vi "_read_LO_params.vi"(10 "Control":T5={"GPIB_ATT"="28", "6501Dev#"=1, "GPIB_SP"="18", "GPIB_PM"="13", "GPIB_DSA"="11", "GPIB_DMM (TPD)"="23", "GPIB_MPI"="2", "mortorÝè"=[{"Axis"=0, "ID"=0, "HIspeed"=200.0, "LOspeed"=100.0, "ACCEL(ms)"=100.0, "Sratio"=50.0, "フリーラン\n"=FALSE, "•¶Žš—ñ"="DSB HOT/COLD"}, {"Axis"=1, "ID"=0, "HIspeed"=4.0, "LOspeed"=4.0, "ACCEL(ms)"=100.0, "Sratio"=50.0, "フリーラン\n"=TRUE, "•¶Žš—ñ"="SubMM Att"}, {"Axis"=0, "ID"=0, "HIspeed"=200.0, "LOspeed"=100.0, "ACCEL(ms)"=100.0, "Sratio"=50.0, "フリーラン\n"=TRUE, "•¶Žš—ñ"="MPI Port1"}, {"Axis"=1, "ID"=0, "HIspeed"=200.0, "LOspeed"=100.0, "ACCEL(ms)"=100.0, "Sratio"=50.0, "フリーラン\n"=TRUE, "•¶Žš—ñ"="MPI Port2"}, {"Axis"=1, "ID"=0, "HIspeed"=200.0, "LOspeed"=100.0, "ACCEL(ms)"=100.0, "Sratio"=50.0, "フリーラン\n"=TRUE, "•¶Žš—ñ"="gainComp"}], "DATAパス"=path "C:/Documents and Settings/?澤佳?/デスクトップ/data/プロトカ?トリッジ/110113_protoC4-9/110127_mixtest", "DBパス "=path "Z:/band10/Labview_ALMA/MIX95/test", "comment"="mix10test", "ColdCarts"="003601", "Th"=300.0, "Tc"=77.0, "Set_SIS_volt"=2.0999999046325684, "Offset"=0.0, "control"=0, "FreqLO"=874.0, "Set_Mag_Cur"=800.0, "MPI offset(mm)"=22.962, "HOT/COLD"=0} {"HOT/COLD" items=["DSB", "SBR (Cart.)", "GainComp", "SBR (MIX)"]; "control" items=["CLOSE LOOP", "OPEN LOOP", "Not Control"]}, 11 "Bias_LO_equip":T7={"Node address"=19, "CAN Interface"="CAN1", "Cartridge band"=10, "Slave Node in"={"Address"=19, "Serial Number"=[16, 71, 55, 76, 1, 8, 0, -15]}, "ObjHandle out"=214106176, "POL"=1, "sb"=1, "GPIB_SM (SIS S,V)"="24", "GPIB_DMM (SIS I)"="22", "GPIB_SM (MAG I) "="25", "GPIB_SG(LO)"="19", "GPIB_PW (PAMP) "="6", "GPIB_TMP1(8ch)"="12", "GPIB_TMP2(2ch)  "="13", "WCA_avg"=10, "Rsen"=10.0, "BiasModule"=1, "LOModule "=5, "WCA_LO_FREQ_SET"={"YTO Low freq. [GHz]"=14.42, "YTO High freq. [GHz]"=17.7, "Kvco"=1, "Lock Pol."=0, "SET LO FREQ"=96.22222, "Multiplier"=6.0, "YTO (HEX)"=2014, "YTO ( FREQ)"=16.033167, "NULL PLL INTEGRATOR"=FALSE}, "Res for"=0} {"Res for" items=["none", "series res", "parallel res"]; "WCA_LO_FREQ_SET"."YTO ( FREQ)" min=25 max=150 step=0.0001 format="%.3f"; "WCA_LO_FREQ_SET"."Multiplier" min=3 max=6 step=3; "WCA_LO_FREQ_SET"."SET LO FREQ" min=25 max=150 step=0.0001 format="%.3f"; "WCA_LO_FREQ_SET"."Lock Pol." items=["Lower", "Upper"]; "WCA_LO_FREQ_SET"."Kvco" items=["7.5MHz/V", "15MHz/V"]; "WCA_LO_FREQ_SET"."YTO High freq. [GHz]" format="%.3f"; "WCA_LO_FREQ_SET"."YTO Low freq. [GHz]" format="%.3f"; "BiasModule" items=["B10Lab Bias"=0, "WCA BiasModule"=1, "none"=99]; "Slave Node in"."Serial Number" format="%.0x"; "Slave Node in"."Address" format="%.0x"; "Cartridge band" max=10 step=1; "Node address" format="%.0x"}) -> (3 "•¶Žš—ñ":string="PreampParam, 3.65, 874.00, 2011-02-04  19:50:11, 1.40, 0.00, 0.00,  12.05, 0.00, 0.02,  -1.53, 4.91, 4.91,")   [LabVIEW 2017]
uses:
  WCA_NAOJ_sub_vi/WCA_Global.vi
panel:
  out "GET_PLL":T1={"PLL_ASSY_T"=37.887573, "PLL_REF_TOT_P"=-0.004119873, "PLL_IF_TOT_P"=0.010223389, "PLL_CORR_V"=0.08273038, "PLL_LOCK_V"=0.06496083, "PLL_5V_SUPPLY_V"=19.049072, "Temp_TF"=TRUE, "PLL Ref Pwr_TF"=FALSE, "IF Pwr_TF"=FALSE, "PLL Corr_TF"=TRUE, "PLL Lock V_TF"=FALSE, "PLL Nominal_TF"=FALSE}
  out "GET_PA":T2={"PA_A_DRAIN_V"=4.0403748, "PA_A_DRAIN_C"=429.99268, "PA_A_GATE_V"=-0.00061035156, "PA_B_DRAIN_V"=0.0048828125, "PA_B_DRAIN_C"=2.5482178, "PA_B_GATE_V"=0.0015258789, "PA_3V_SUPPLY_V"=3.7130737, "PA_5V_MON"=5.3082275}
  out "GET_AMC":T3={"AMC_A_DRAIN_V"=3.48938, "AMC_A_DRAIN_C"=64.42261, "AMC_A_GATE_V"=-0.4689026, "AMC_B_DRAIN_V"=4.34021, "AMC_B_DRAIN_C"=301.4679, "AMC_B_GATE_V"=-0.48934937, "AMC_E_DRAIN_V"=3.977356, "AMC_E_DRAIN_C"=342.6819, "AMC_E_GATE_V"=-0.24169922, "AMC_3V_SUPPLY_V"=-13.227844, "AMC_5V_MON"=5.204468, "AMC_MULT_D_V"=0.0}
  out "GET_PHOTOMIXER":T4={"PHOTMIX_ State"=enum."Disabled", "PHOTOMIX_BIAS_V"=-0.0012207031, "PHOTOMIX_BIAS_C"=-0.0032043457}
  in  "CLNA_SET":T6={"CLNA State"=1, "SET POL0 LNA1 STAGE1 DRAIN V"=0.0, "SET POL0 LNA1 STAGE1 DRAIN C"=0.0, "SET POL0 LNA1 STAGE2 DRAIN V"=0.0, "SET POL0 LNA1 STAGE2 DRAIN C"=0.0, "SET POL0 LNA1 STAGE3 DRAIN V"=0.0, "SET POL0 LNA1 STAGE3 DRAIN C"=0.0} {"SET POL0 LNA1 STAGE3 DRAIN C" min=0 max=20 step=0.01 format="%.2f"; "SET POL0 LNA1 STAGE3 DRAIN V" min=0 max=3 step=0.01 format="%.2f"; "SET POL0 LNA1 STAGE2 DRAIN C" min=0 max=20 step=0.01 format="%.2f"; "SET POL0 LNA1 STAGE2 DRAIN V" min=0 max=3 step=0.01 format="%.2f"; "SET POL0 LNA1 STAGE1 DRAIN C" min=0 max=20 step=0.01 format="%.2f"; "SET POL0 LNA1 STAGE1 DRAIN V" min=0 max=3 step=0.01 format="%.2f"; "CLNA State" items=["Disabled", "Enabled"]}
  out "Link済み":bool
  # "Vd [V]"
  # "Id [mA]"
  # "Vg [V]"
  # "PA -3V Supply"
  # "PA A"
  # "-3V"
  # "PA B"
  # "+5V"
  # "Vd [V]"
  # "Id [mA]"
  # "Vg [V]"
  # "AMC A"
  # "AMC B"
  # "AMC E"
  # "Vd [V]"
  # "Id [mA]"
  # "Stage 1"
  # "Stage 2"
  # "Stage 3"
  # "LO freq. [GHz]"
  # "YTO LOW\n/High Freq."
  # "ZERO Intgrtr"
  # "Node Address"
  # "Serial Number"
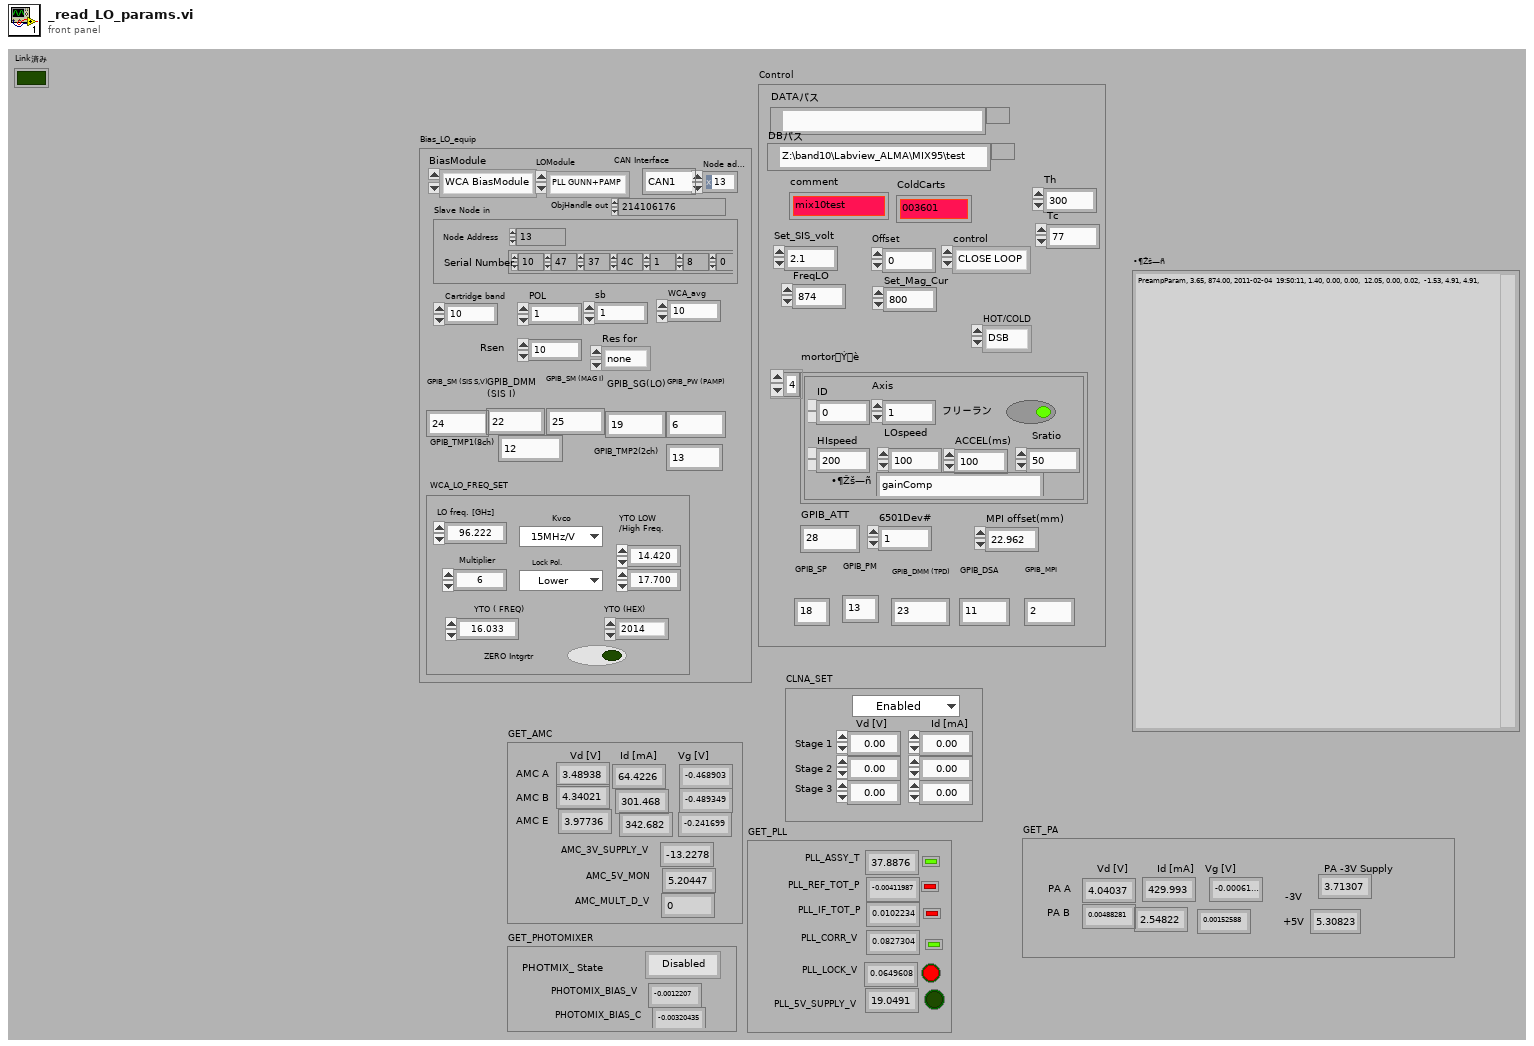
[diagram p1: front panel]
types:
  T1 = cluster{"PLL_ASSY_T":sgl, "PLL_REF_TOT_P":sgl, "PLL_IF_TOT_P":sgl, "PLL_CORR_V":sgl, "PLL_LOCK_V":sgl, "PLL_5V_SUPPLY_V":sgl, "Temp_TF":bool, "PLL Ref Pwr_TF":bool, "IF Pwr_TF":bool, "PLL Corr_TF":bool, "PLL Lock V_TF":bool, "PLL Nominal_TF":bool}
  T2 = cluster{"PA_A_DRAIN_V":sgl, "PA_A_DRAIN_C":sgl, "PA_A_GATE_V":sgl, "PA_B_DRAIN_V":sgl, "PA_B_DRAIN_C":sgl, "PA_B_GATE_V":sgl, "PA_3V_SUPPLY_V":sgl, "PA_5V_MON":sgl}
  T3 = cluster{"AMC_A_DRAIN_V":sgl, "AMC_A_DRAIN_C":sgl, "AMC_A_GATE_V":sgl, "AMC_B_DRAIN_V":sgl, "AMC_B_DRAIN_C":sgl, "AMC_B_GATE_V":sgl, "AMC_E_DRAIN_V":sgl, "AMC_E_DRAIN_C":sgl, "AMC_E_GATE_V":sgl, "AMC_3V_SUPPLY_V":sgl, "AMC_5V_MON":sgl, "AMC_MULT_D_V":sgl}
  T4 = cluster{"PHOTMIX_ State":enum16{"Disabled", "Enabled"}, "PHOTOMIX_BIAS_V":sgl, "PHOTOMIX_BIAS_C":sgl}
  T5 = cluster{"GPIB_ATT":string, "6501Dev#":i16, "GPIB_SP":string, "GPIB_PM":string, "GPIB_DSA":string, "GPIB_DMM (TPD)":string, "GPIB_MPI":string, "mortorÝè":cluster{"Axis":i16, "ID":i16, "HIspeed":dbl, "LOspeed":dbl, "ACCEL(ms)":dbl, "Sratio":dbl, "フリーラン\n":bool, "•¶Žš—ñ":string}[], "DATAパス":path, "DBパス ":path, "comment":string, "ColdCarts":string, "Th":dbl, "Tc":dbl, "Set_SIS_volt":dbl, "Offset":dbl, "control":u16, "FreqLO":dbl, "Set_Mag_Cur":dbl, "MPI offset(mm)":dbl, "HOT/COLD":u16}
  T6 = cluster{"CLNA State":u8, "SET POL0 LNA1 STAGE1 DRAIN V":sgl, "SET POL0 LNA1 STAGE1 DRAIN C":sgl, "SET POL0 LNA1 STAGE2 DRAIN V":sgl, "SET POL0 LNA1 STAGE2 DRAIN C":sgl, "SET POL0 LNA1 STAGE3 DRAIN V":sgl, "SET POL0 LNA1 STAGE3 DRAIN C":sgl}
  T7 = cluster{"Node address":u16, "CAN Interface":string, "Cartridge band":u32, "Slave Node in":cluster{"Address":i16, "Serial Number":i8[]}, "ObjHandle out":u32, "POL":u32, "sb":u32, "GPIB_SM (SIS S,V)":string, "GPIB_DMM (SIS I)":string, "GPIB_SM (MAG I) ":string, "GPIB_SG(LO)":string, "GPIB_PW (PAMP) ":string, "GPIB_TMP1(8ch)":string, "GPIB_TMP2(2ch)  ":string, "WCA_avg":i32, "Rsen":dbl, "BiasModule":u16, "LOModule ":u16, "WCA_LO_FREQ_SET":cluster{"YTO Low freq. [GHz]":sgl, "YTO High freq. [GHz]":sgl, "Kvco":u16, "Lock Pol.":u16, "SET LO FREQ":sgl, "Multiplier":sgl, "YTO (HEX)":u16, "YTO ( FREQ)":sgl, "NULL PLL INTEGRATOR":bool}, "Res for":u16}
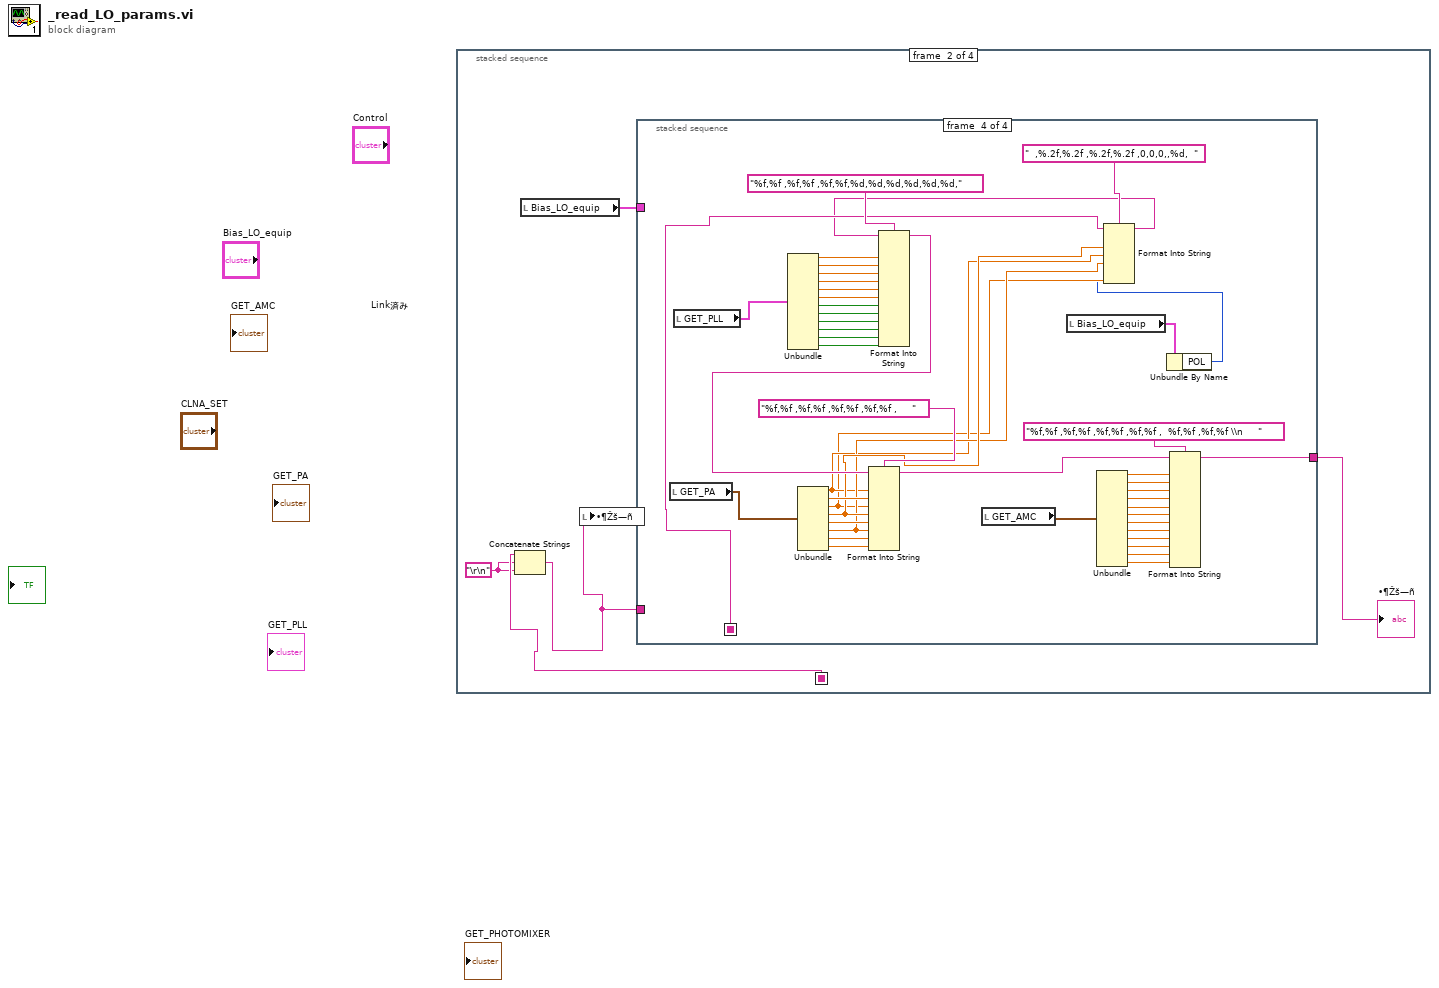
[diagram p0: block diagram]
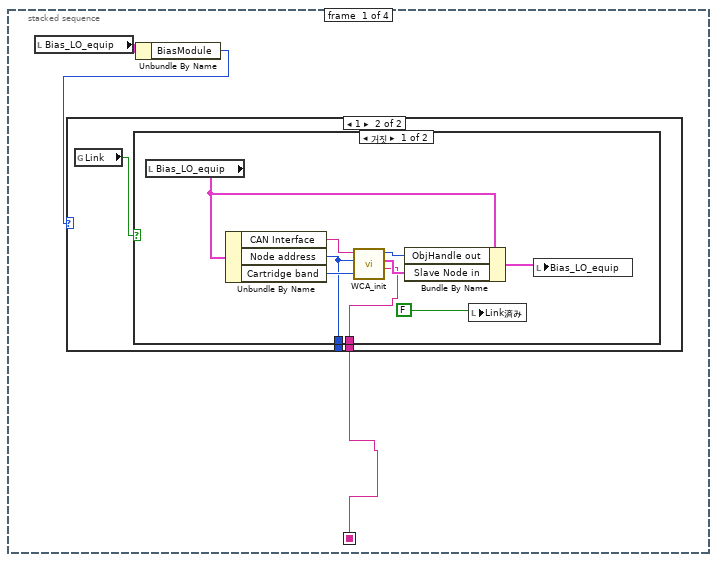
[diagram p2: hidden frame]
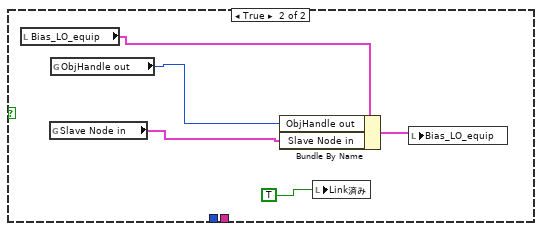
[diagram p4: hidden frame]
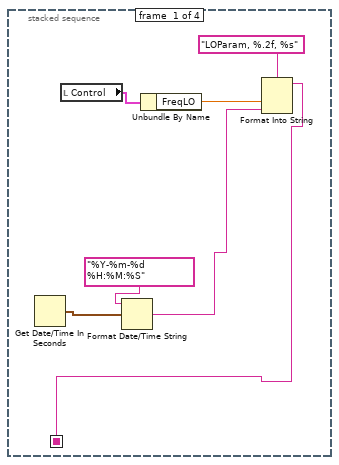
[diagram p5: hidden frame]
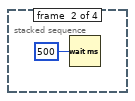
[diagram p6: hidden frame]
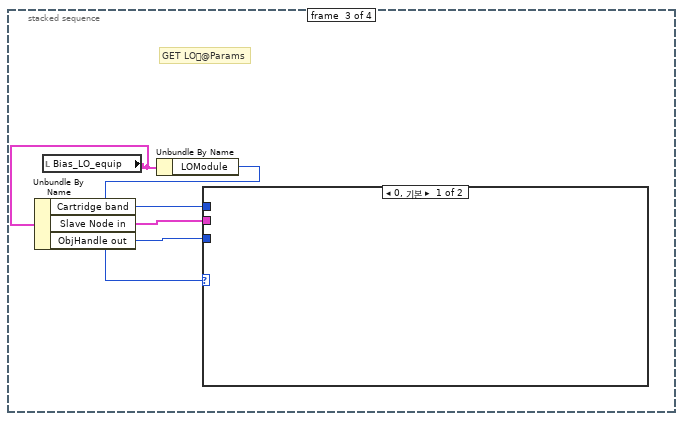
[diagram p7: hidden frame]
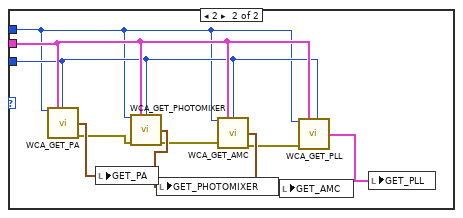
[diagram p8: hidden frame]
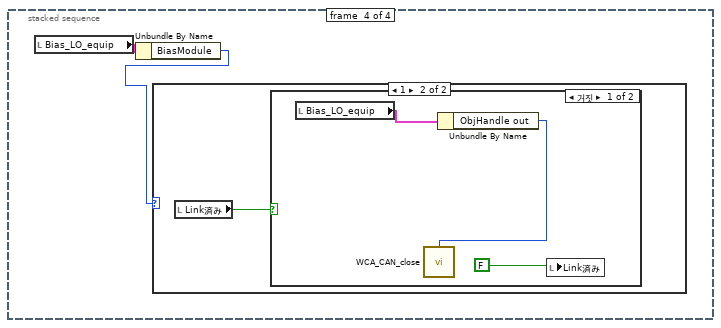
[diagram p10: hidden frame]
diagram:
  n1 = stacked-sequence {
    seq-local: [w1 _ _ _] -> [_ w25 _ _]
    frame #0 {
      n2 = local read "Bias_LO_equip"() -> (w3:T7)
      n3 = Unbundle By Name(w3) -> ("BiasModule"=w2:u16)
      n4 = case shown="1" w2 {
        tunnel: [_ w5] -> w1
        tunnel: [_ w4] -> _
        frame 0, Default {
        }
        frame 1 {
          n5 = global read "WCA_Global.vi" "Link"() -> (w6:bool)
          n6 = case shown="거짓" w6 {
            tunnel: [w7 _] -> w5
            tunnel: [w8 _] -> w4
            frame False {
              n7 = local read "Bias_LO_equip"() -> (w9:T7)
              n8 = Unbundle By Name(w9) -> ("CAN Interface"=w12:string, "Node address"=w8:u16, "Cartridge band"=w11:u32)
              n9 = call "WCA_init.vi"("Cartridge band"=w11, "Node address"=w8, "CAN Interface"=w12) -> ("Detected CAN Nodes."=w7:string, "Slave Node in"=w14:cluster{"Address":i16, "Serial Number":i8[]}, "ObjHandle out"=w15:u32)  [unwired: 4 in, 2 out]
              n10 = Bundle By Name(cluster=w9, "ObjHandle out"=w15, "Slave Node in"=w14) -> (w10:T7)
              n11 = local write "Link済み"(FALSE) -> ()
              n12 = local write "Bias_LO_equip"(w10) -> ()
            }
            frame True {
              n13 = local read "Bias_LO_equip"() -> (w19:T7)
              n14 = global read "WCA_Global.vi" "Slave Node in"() -> (w17:cluster{"Address":i16, "Serial Number":i8[]})
              n15 = global read "WCA_Global.vi" "ObjHandle out"() -> (w18:u32)
              n16 = Bundle By Name(cluster=w19, "ObjHandle out"=w18, "Slave Node in"=w17) -> (w20:T7)
              n17 = local write "Link済み"(TRUE) -> ()
              n18 = local write "Bias_LO_equip"(w20) -> ()
            }
          }
        }
      }
    }
    frame #1 {
      w24 = "\r\n"
      n19 = Concatenate Strings(w25, w24, w24) -> (w23:string)
      n20 = local read "Bias_LO_equip"() -> (w22:T7)
      n21 = local write "•¶Žš—ñ"(w23) -> ()
      n22 = stacked-sequence {
        seq-local: [w26 _ _ _] -> [_ _ _ w60]
        tunnel: w23 -> [_ _ _ _]
        tunnel: w22 -> [_ _ _ _]
        tunnel: [_ _ _ w55] -> w21
        frame #0 {
          n23 = Get Date/Time In Seconds() -> (seconds since 1Jan1904=w31:timestamp)
          n24 = local read "Control"() -> (w29:T5)
          n25 = Format Date/Time String(time format string (%c)="%Y-%m-%d  %H:%M:%S", seconds (now)=w31) -> (date/time string=w27:string)  [unwired: 1 in]
          n26 = Unbundle By Name(w29) -> ("FreqLO"=w28:dbl)
          n27 = Format Into String(format string="LOParam, %.2f, %s", w28, w27) -> (resulting string=w26:string)  [unwired: 2 in, 1 out]
        }
        frame #1 {
          n28 = Wait (ms)(milliseconds to wait=500) -> ()  [unwired: 1 out]
        }
        frame #2 {
          # "GET LO@Params"
          n29 = local read "Bias_LO_equip"() -> (w34:T7)
          n30 = Unbundle By Name(w34) -> ("Cartridge band"=w37:u32, "Slave Node in"=w36:cluster{"Address":i16, "Serial Number":i8[]}, "ObjHandle out"=w35:u32)
          n31 = Unbundle By Name(w34) -> ("LOModule"=w38:u16)
          n32 = case shown="0, 기본" w38 {
            tunnel: w36 -> [_ w44]
            tunnel: w35 -> [_ w43]
            tunnel: w37 -> [_ w42]
            frame 0, Default {
            }
            frame 2 {
              n33 = call "WCA_GET_PA.vi"("Cartridge Band"=w42, "Slave Node in"=w44, "ObjHandle in"=w43) -> ("GET_PA"=w45:T2, "error out"=w41:errorcluster)  [unwired: 10 in, 1 out]
              n34 = local write "GET_PA"(w45) -> ()
              n35 = call "WCA_GET_PHOTOMIXER.vi"("Cartridge Band"=w42, "Slave Node in"=w44, "ObjHandle in"=w43, "error in (no error)"=w41) -> ("GET_PHOTOMIXER"=w47:T4, "error out"=w40:errorcluster)  [unwired: 9 in, 1 out]
              n36 = local write "GET_PHOTOMIXER"(w47) -> ()
              n37 = call "WCA_GET_AMC.vi"("Cartridge Band"=w42, "Slave Node in"=w44, "ObjHandle in"=w43, "error in (no error)"=w40) -> ("GET_AMC"=w48:T3, "error out"=w39:errorcluster)  [unwired: 9 in, 1 out]
              n38 = local write "GET_AMC"(w48) -> ()
              n39 = call "WCA_GET_PLL.vi"("Cartridge Band"=w42, "Slave Node in"=w44, "ObjHandle in"=w43, "error in (no error)"=w39) -> ("GET_PLL"=w46:T1)  [unwired: 9 in, 2 out]
              n40 = local write "GET_PLL"(w46) -> ()
            }
          }
        }
        frame #3 {
          n41 = local read "GET_PA"() -> (w66:T2)
          n42 = local read "GET_PLL"() -> (w93:T1)
          n43 = Unbundle(w93) -> ("PLL_ASSY_T"=w92:sgl, "PLL_REF_TOT_P"=w91:sgl, "PLL_IF_TOT_P"=w90:sgl, "PLL_CORR_V"=w89:sgl, "PLL_LOCK_V"=w88:sgl, "PLL_5V_SUPPLY_V"=w87:sgl, "Temp_TF"=w86:bool, "PLL Ref Pwr_TF"=w85:bool, "IF Pwr_TF"=w84:bool, "PLL Corr_TF"=w83:bool, "PLL Lock V_TF"=w82:bool, "PLL Nominal_TF"=w81:bool)
          n44 = Unbundle(w66) -> ("PA_A_DRAIN_V"=w52:sgl, "PA_A_DRAIN_C"=w65:sgl, "PA_A_GATE_V"=w51:sgl, "PA_B_DRAIN_V"=w54:sgl, "PA_B_DRAIN_C"=w64:sgl, "PA_B_GATE_V"=w53:sgl, "PA_3V_SUPPLY_V"=w63:sgl, "PA_5V_MON"=w62:sgl)
          n45 = local read "GET_AMC"() -> (w80:T3)
          n46 = local read "Bias_LO_equip"() -> (w50:T7)
          n47 = Unbundle(w80) -> ("AMC_A_DRAIN_V"=w79:sgl, "AMC_A_DRAIN_C"=w78:sgl, "AMC_A_GATE_V"=w77:sgl, "AMC_B_DRAIN_V"=w76:sgl, "AMC_B_DRAIN_C"=w74:sgl, "AMC_B_GATE_V"=w75:sgl, "AMC_E_DRAIN_V"=w73:sgl, "AMC_E_DRAIN_C"=w72:sgl, "AMC_E_GATE_V"=w71:sgl, "AMC_3V_SUPPLY_V"=w70:sgl, "AMC_5V_MON"=w69:sgl, "AMC_MULT_D_V"=w68:sgl)
          n48 = Unbundle By Name(w50) -> ("POL"=w49:u32)
          n49 = Format Into String(format string="  ,%.2f,%.2f ,%.2f,%.2f ,0,0,0,,%d,  ", initial string=w60, w54, w52, w53, w51, w49) -> (resulting string=w58:string)  [unwired: 1 in, 1 out]
          n50 = Format Into String(format string="%f,%f ,%f,%f ,%f,%f,%d,%d,%d,%d,%d,%d,", initial string=w58, w92, w91, w90, w89, w88, w87, w86, w85, w84, w83, w82, w81) -> (resulting string=w57:string)  [unwired: 1 in, 1 out]
          n51 = Format Into String(format string="%f,%f ,%f,%f ,%f,%f ,%f,%f ,     ", initial string=w57, w52, w65, w51, w54, w64, w53, w63, w62) -> (resulting string=w56:string)  [unwired: 1 in, 1 out]
          n52 = Format Into String(format string="%f,%f ,%f,%f ,%f,%f ,%f,%f ,  %f,%f ,%f,%f \\n     ", initial string=w56, w79, w78, w77, w76, w74, w75, w73, w72, w71, w70, w69, w68) -> (resulting string=w55:string)  [unwired: 1 in, 1 out]
        }
      }
      "•¶Žš—ñ" <- w21
    }
    frame #2 {
    }
    frame #3 {
      n53 = local read "Bias_LO_equip"() -> (w96:T7)
      n54 = Unbundle By Name(w96) -> ("BiasModule"=w95:u16)
      n55 = case shown="1" w95 {
        frame 0, Default {
        }
        frame 1 {
          n56 = local read "Link済み"() -> (w97:bool)
          n57 = case shown="거짓" w97 {
            frame False {
              n58 = local read "Bias_LO_equip"() -> (w99:T7)
              n59 = Unbundle By Name(w99) -> ("ObjHandle out"=w98:u32)
              n60 = call "WCA_CAN_close.vi"("ObjHandle in"=w98) -> ()  [unwired: 14 in, 1 out]
              n61 = local write "Link済み"(FALSE) -> ()
            }
            frame True {
            }
          }
        }
      }
    }
  }
